vi "SHO diffEQ.vi"(2 "data":variant, 3 "t":dbl, 4 "x":dbl[](array[numeric])) -> (0 "error out":errorcluster, 1 "f(x,t)":dbl[](array[numeric]))   [LabVIEW 2015]
doc: "This template is the starting point for creating a function that is the right-hand-side of an ordinary differential equaltion to be passed to the ODE Solver.vi."
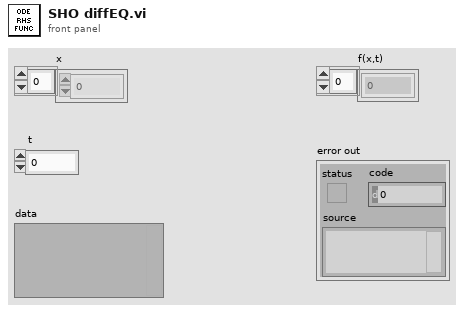
[diagram p1: front panel]
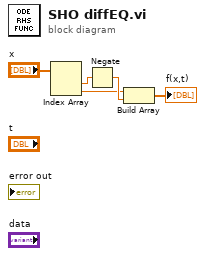
[diagram p0: block diagram]
diagram:
  n1 = Index Array(array="x") -> (element #1=w4:dbl, element #2=w2:dbl)  [unwired: 2 in]
  n2 = Negate(x=w4) -> (-x=w3:dbl)
  n3 = Build Array(w2, w3) -> (→"f(x,t)":dbl[])
